vi "Init images and strings.vi"(8 "error in (no error)":errorcluster, 10 "Image ref array":refnum<vi>[](array[refnum]), 11 "Label array":refnum<vi>[](array[refnum])) -> (0 "error in (no error) 2":errorcluster)   [LabVIEW 2019, in "ZenGage v3.0 UI.lvclass"]
uses:
  ZenGage v3.0 UI.lvclass
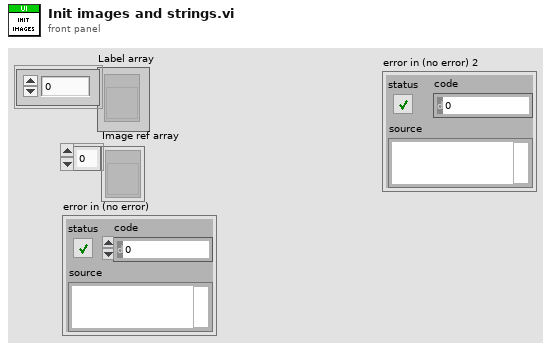
[diagram p1: front panel]
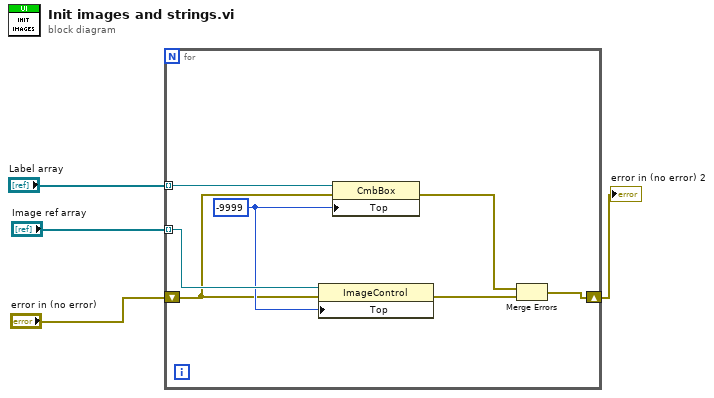
[diagram p0: block diagram]
diagram:
  n1 = for {
    tunnel: "Label array" -> [w11] mode=indexing
    tunnel: "Image ref array" -> [w10] mode=indexing
    shift-right: [w7] -> w1
    shift-left: "error in (no error)" -> [w5]
    w6 = -9999 ("Position:Top")
    n2 = property class="ImageControl"(reference=w10, error in=w5, "Top"=w6) -> (error out=w9:errorcluster)  [unwired: 1 out]
    n3 = property class="CmbBox"(reference=w11, error in=w5, "Top"=w6) -> (error out=w8:errorcluster)  [unwired: 1 out]
    n4 = Merge Errors(w8, w9) -> (w7:errorcluster)
  }
  "error in (no error) 2" <- w1
